vi "DetectColor.vi"() -> (3 "Color":T1=enum."Yellow")   [LabVIEW 2019]
uses:
  Controls/Colors.ctl
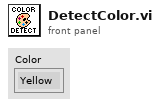
[diagram p1: front panel]
types:
  T1 = typedef "Colors.ctl" = enum16{"Unknown", "Yellow", "Red", "Green", "Blue"}
  T2 = typedef "Color Sensor V3 DevRef.ctl" = cluster{"I2CDevRef":T3}
  T3 = typedef "WPI_I2CDevRef.ctl" = cluster{"DevStatus":errorcluster, "Device Address":u8, "Handle":i32, "I2C Bus":T4}
  T4 = typedef "i2c_bus.ctl" = enum16{"I2C On-Board", "I2C MXP", "Invalid"}
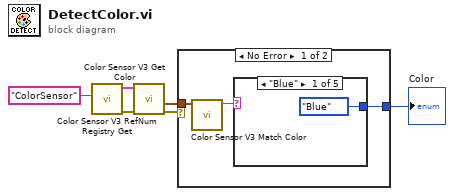
[diagram p0: block diagram]
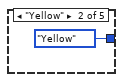
[diagram p2: hidden frame]
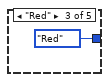
[diagram p3: hidden frame]
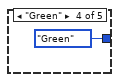
[diagram p4: hidden frame]
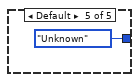
[diagram p5: hidden frame]
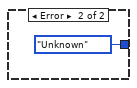
[diagram p6: hidden frame]
diagram:
  n1 = call <vilib>:"Color Sensor V3 RefNum Registry Get.vi"("refnum name"="ColorSensor") -> ("error out"=w2:errorcluster, "ColorSensorDevRef"=w5:T2)  [unwired: 9 in]
  n2 = call <vilib>:"Color Sensor V3 Get Color.vi"("error in (no error)"=w2, "ColorSensorDevRef"=w5) -> ("error out"=w1:errorcluster, "Normalized Color"=w4:cluster{"R":dbl, "G":dbl, "B":dbl})  [unwired: 6 in, 2 out]
  n3 = case shown="No Error" w1 {
    tunnel: w4 -> [w9 _]
    tunnel: [w7 Colors."Unknown" ("Color")] -> w3
    frame No Error {
      n4 = call <vilib>:"Color Sensor V3 Match Color.vi"("Measured Color"=w9) -> ("Matched Color Name"=w8:string)  [unwired: 8 in, 2 out]
      n5 = case shown="\"Blue\"" w8 {
        tunnel: [Colors."Blue" ("Color 2") Colors."Yellow" ("Color") Colors."Red" ("Color") Colors."Green" ("Color") Colors."Unknown" ("Color")] -> w7
        frame "Blue" {
        }
        frame "Yellow" {
        }
        frame "Red" {
        }
        frame "Green" {
        }
        frame Default {
        }
      }
    }
    frame Error {
    }
  }
  "Color" <- w3
